vi "Read UI Constants.vi"(8 "error in (no error)":errorcluster, 11 "CFG File Refnum in":T2) -> (0 "error out":errorcluster, 2 "MHL Configuration":T1, 3 "refnum out":T2)   [LabVIEW 2017]
uses:
  <vilib>/Utility/config.llb/Config Data RefNum.ctl
  controls/MHL Configuration.ctl
  Boiler System Globals.vi
  <vilib>/Utility/config.llb/Read Key (Double).vi
  <vilib>/Utility/error.llb/Error Cluster From Error Code.vi
  <vilib>/ErrorRing/Error Ring.xnode
  <vilib>/Utility/config.llb/NI_LVConfig.lvlib
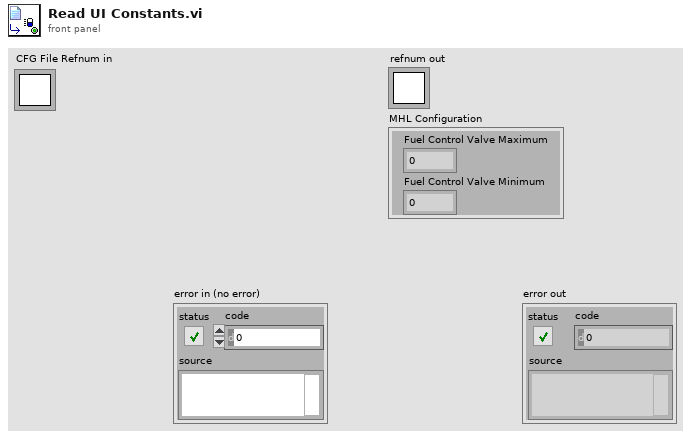
[diagram p1: front panel]
types:
  T1 = typedef "MHL Configuration.ctl" = cluster{"Fuel Control Valve Maximum":dbl, "Fuel Control Valve Minimum":dbl}
  T2 = typedef "NI_LVConfig.lvlib/Config Data RefNum.ctl" = refnum<k1>
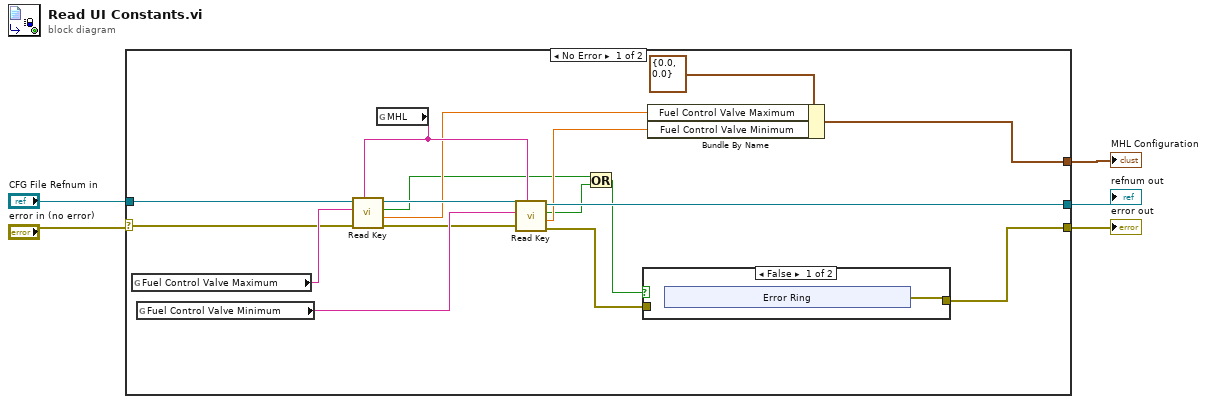
[diagram p0: block diagram]
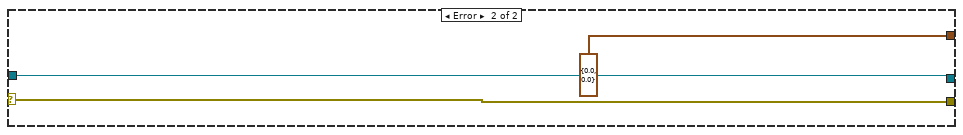
[diagram p3: hidden frame]
diagram:
  n1 = case shown="No Error" "error in (no error)" {
    selector: "error in (no error)" -> [w12 w30]
    tunnel: "CFG File Refnum in" -> [w21 w31]
    tunnel: [w17 w31] -> w3
    tunnel: [w13 T1 {"Fuel Control Valve Maximum"=0.0, "Fuel Control Valve Minimum"=0.0} ("MHL Configuration")] -> w2
    tunnel: [w7 w30] -> w1
    frame No Error {
      n2 = global read "Boiler System Globals.vi" "Fuel Control Valve Maximum"() -> (w20:string)
      n3 = global read "Boiler System Globals.vi" "Fuel Control Valve Minimum"() -> (w19:string)
      n4 = global read "Boiler System Globals.vi" "MHL"() -> (w22:string)
      n5 = call-poly <vilib>:"Read Key.vi"("section"=w22, "error in (no error)"=w12, "key"=w20, "refnum"=w21) -> ("error out"=w11:errorcluster, "value"=w15:dbl, "found?"=w9:bool, "refnum out"=w18:T2)  [unwired: 4 in]
      n6 = call-poly <vilib>:"Read Key.vi"("section"=w22, "error in (no error)"=w11, "key"=w19, "refnum"=w18) -> ("error out"=w8:errorcluster, "value"=w14:dbl, "found?"=w10:bool, "refnum out"=w17:T2)  [unwired: 4 in]
      n7 = Or(x=w9, y=w10) -> (x .or. y?=w6:bool)
      n8 = case shown="False" w6 {
        tunnel: w8 -> [_ w29]
        tunnel: [w23 w29] -> w7
        frame False {
          n9 = xnode "Error Ring"() -> ("error out"=w23:errorcluster)
        }
        frame True {
        }
      }
      n10 = Bundle By Name(cluster=T1 {"Fuel Control Valve Maximum"=0.0, "Fuel Control Valve Minimum"=0.0} ("MHL Configuration"), "Fuel Control Valve Maximum"=w15, "Fuel Control Valve Minimum"=w14) -> (w13:T1)
    }
    frame Error {
    }
  }
  "error out" <- w1
  "refnum out" <- w3
  "MHL Configuration" <- w2
